vi "Message to Array.vi"(0 "reference in":refnum<class "Result Logger.lvclass">, 4 "Messages":T1[](array[typedef]), 5 "error in (no error)":errorcluster) -> (14 "reference out":refnum<class "Result Logger.lvclass">, 18 "Test Result Array":string[][](array[string]), 19 "error out":errorcluster)   [LabVIEW 2017, in "Result Logger.lvclass"]
uses:
  Result Logger.lvclass
  public/Message.ctl
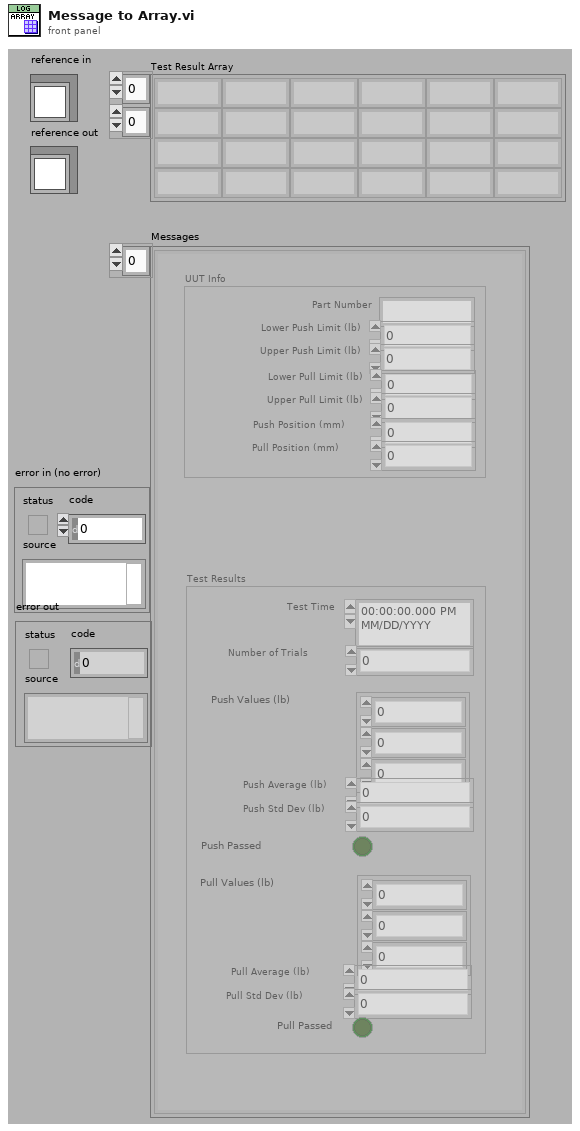
[diagram p1: front panel]
types:
  T1 = typedef "Result Logger.lvclass/Message.ctl" = cluster{"UUT Info":cluster{"Part Number":string, "Lower Push Limit (lb)":dbl, "Upper Push Limit (lb)":dbl, "Lower Pull Limit (lb)":dbl, "Upper Pull Limit (lb)":dbl, "Push Position (mm)":dbl, "Pull Position (mm)":dbl}, "Test Results":cluster{"Test Time":timestamp, "Number of Trials":u32, "Push Values (lb)":dbl[], "Push Average (lb)":dbl, "Push Std Dev (lb)":dbl, "Push Passed":bool, "Pull Values (lb)":dbl[], "Pull Average (lb)":dbl, "Pull Std Dev (lb)":dbl, "Pull Passed":bool}}
  T2 = cluster{"Part Number":string, "Lower Push Limit (lb)":dbl, "Upper Push Limit (lb)":dbl, "Lower Pull Limit (lb)":dbl, "Upper Pull Limit (lb)":dbl, "Push Position (mm)":dbl, "Pull Position (mm)":dbl}
  T3 = cluster{"Test Time":timestamp, "Number of Trials":u32, "Push Values (lb)":dbl[], "Push Average (lb)":dbl, "Push Std Dev (lb)":dbl, "Push Passed":bool, "Pull Values (lb)":dbl[], "Pull Average (lb)":dbl, "Pull Std Dev (lb)":dbl, "Pull Passed":bool}
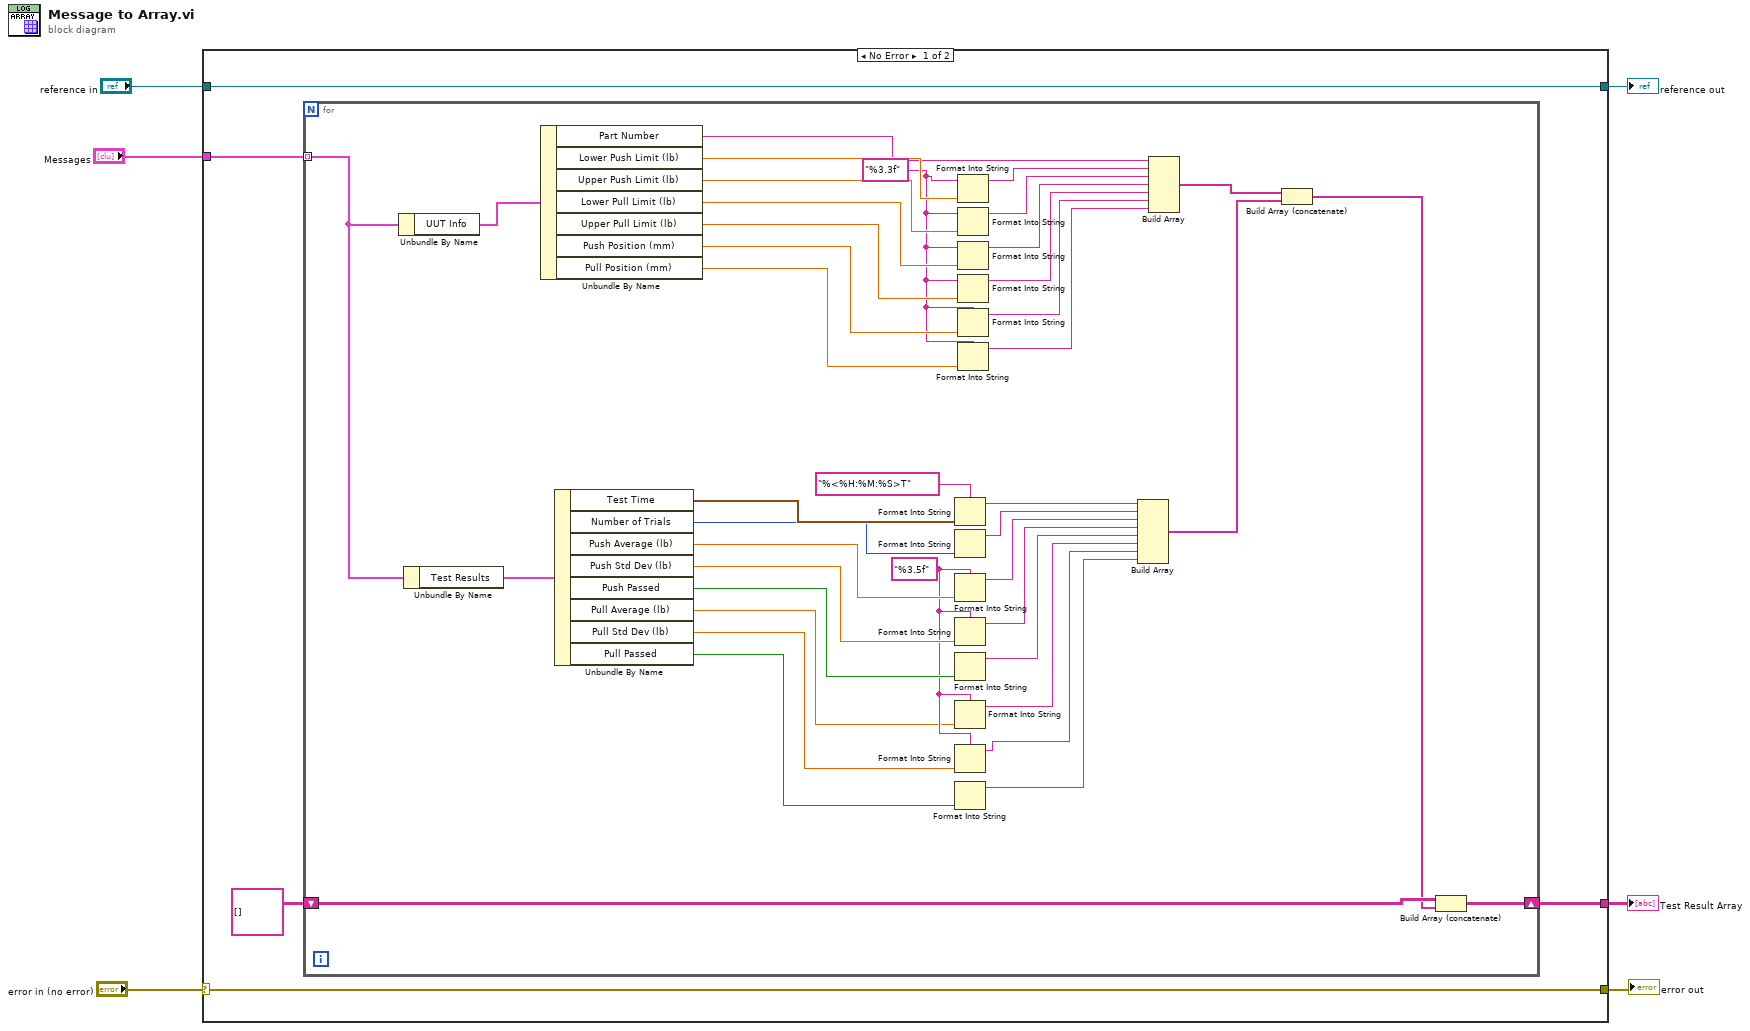
[diagram p0: block diagram]
diagram:
  n1 = case shown="No Error" "error in (no error)" {
    selector: "error in (no error)" -> [w10 w53]
    tunnel: [w10 w53] -> w5
    tunnel: [w11 w52] -> w3
    tunnel: "reference in" -> [w11 w52]
    tunnel: "Messages" -> [w9 _]
    tunnel: [w8 _] -> w2
    frame No Error {
      n2 = for {
        tunnel: w9 -> [w50] mode=indexing
        shift-right: [w12] -> w8
        shift-left: string[][] [] -> [w51]
        w34 = "%3.5f" ("format string")
        w42 = "%3.3f" ("format string")
        n3 = Unbundle By Name(w50) -> ("UUT Info"=w49:T2)
        n4 = Unbundle By Name(w50) -> ("Test Results"=w41:T3)
        n5 = Unbundle By Name(w49) -> ("Part Number"=w30:string, "Lower Push Limit (lb)"=w48:dbl, "Upper Push Limit (lb)"=w47:dbl, "Lower Pull Limit (lb)"=w46:dbl, "Upper Pull Limit (lb)"=w45:dbl, "Push Position (mm)"=w44:dbl, "Pull Position (mm)"=w43:dbl)
        n6 = Unbundle By Name(w41) -> ("Test Time"=w39:timestamp, "Number of Trials"=w38:u32, "Push Average (lb)"=w37:dbl, "Push Std Dev (lb)"=w36:dbl, "Push Passed"=w35:bool, "Pull Average (lb)"=w33:dbl, "Pull Std Dev (lb)"=w32:dbl, "Pull Passed"=w31:bool)
        n7 = Format Into String(format string="%<%H:%M:%S>T", w39) -> (resulting string=w23:string)  [unwired: 2 in, 1 out]
        n8 = Format Into String(w38) -> (resulting string=w22:string)  [unwired: 3 in, 1 out]
        n9 = Format Into String(format string=w34, w37) -> (resulting string=w21:string)  [unwired: 2 in, 1 out]
        n10 = Format Into String(format string=w34, w36) -> (resulting string=w20:string)  [unwired: 2 in, 1 out]
        n11 = Format Into String(w35) -> (resulting string=w19:string)  [unwired: 3 in, 1 out]
        n12 = Format Into String(format string=w34, w33) -> (resulting string=w18:string)  [unwired: 2 in, 1 out]
        n13 = Format Into String(format string=w34, w32) -> (resulting string=w17:string)  [unwired: 2 in, 1 out]
        n14 = Format Into String(w31) -> (resulting string=w16:string)  [unwired: 3 in, 1 out]
        n15 = Format Into String(format string=w42, w48) -> (resulting string=w29:string)  [unwired: 2 in, 1 out]
        n16 = Format Into String(format string=w42, w47) -> (resulting string=w28:string)  [unwired: 2 in, 1 out]
        n17 = Format Into String(format string=w42, w46) -> (resulting string=w27:string)  [unwired: 2 in, 1 out]
        n18 = Format Into String(format string=w42, w45) -> (resulting string=w26:string)  [unwired: 2 in, 1 out]
        n19 = Format Into String(format string=w42, w44) -> (resulting string=w25:string)  [unwired: 2 in, 1 out]
        n20 = Format Into String(format string=w42, w43) -> (resulting string=w24:string)  [unwired: 2 in, 1 out]
        n21 = Build Array(w23, w22, w21, w20, w19, w18, w17, w16) -> (w14:string[])
        n22 = Build Array(w30, w29, w28, w27, w26, w25, w24) -> (w15:string[])
        n23 = Build Array (concatenate)(w15, w14) -> (w13:string[])
        n24 = Build Array (concatenate)(w51, w13) -> (w12:string[][])
      }
    }
    frame Error {
    }
  }
  "error out" <- w5
  "reference out" <- w3
  "Test Result Array" <- w2
